vi "Project Target Application.vi"(8 "Error In":errorcluster, 10 "Project Name":string, 11 "App In":refnum<vi>) -> (0 "Error Out":errorcluster, 2 "Project Target App":refnum<vi>, 3 "App Out":refnum<vi>)   [LabVIEW 2017, in "Bookmark Manager.lvlib"]
uses:
  Bookmark Manager.lvlib
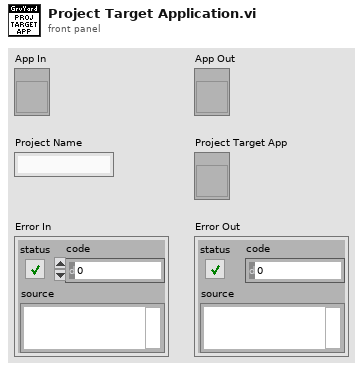
[diagram p1: front panel]
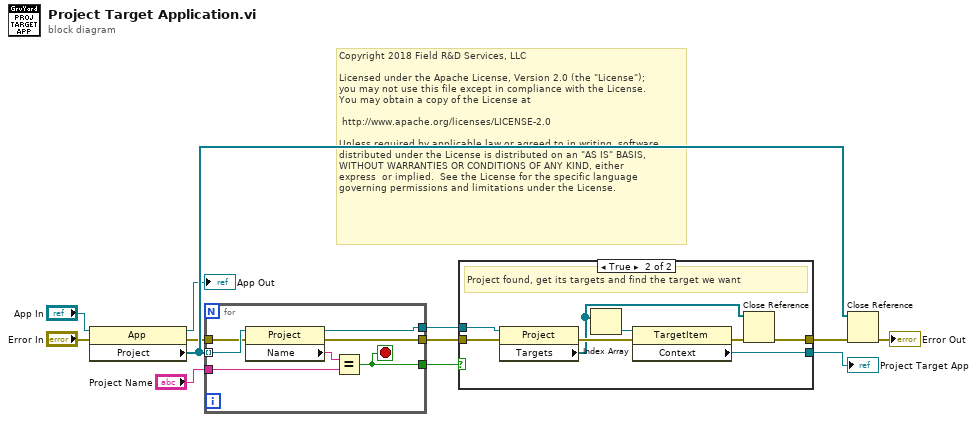
[diagram p0: block diagram]
diagram:
  # "Copyright 2018 Field R&D Services, LLC\n\nLicensed under the Apache License, Version 2.0 (the \"License\");\nyou may not use this file except in compliance with the License.\nYou may obtain a copy of the License at\n\n\thttp://www.apache.org/licenses/LICENSE-2.0\n\nUnless required by applicable law or agreed to in writing, software\ndistributed under the License is distributed on an \"AS IS\" BASIS,\nWITHOUT WARRANTIES OR CONDITIONS OF ANY KIND, either \nexpress  or implied.  See the License for the specific language \ngoverning permissions and limitations under the License."
  n1 = property class="App"(reference="App In", error in="Error In") -> (reference out=→"App Out":refnum<vi>, error out=w5:errorcluster, "Project"=w12:refnum<vi>[])
  n2 = for {
    tunnel: w12 -> [w19] mode=indexing
    tunnel: w5 -> [w18]
    tunnel: "Project Name" -> [w16]
    tunnel: [w15] -> w9
    tunnel: [w14] -> w8
    tunnel: [w13] -> w7
    stop <- w13 stop-if-true
    n3 = property class="Project"(reference=w19, error in=w18) -> (reference out=w15:refnum<vi>, error out=w14:errorcluster, "Name"=w17:string)
    n4 = Equal?(x=w17, y=w16) -> (x = y?=w13:bool)
  }
  n5 = case shown="True" w7 {
    tunnel: w8 -> [w20 w28]
    tunnel: [w20 w22] -> w10
    tunnel: w9 -> [_ w27]
    tunnel: [_ w24] -> w2
    frame False {
      # "Project not found, weird"
    }
    frame True {
      # "Project found, get its targets and find the target we want"
      n6 = property class="Project"(reference=w27, error in=w28) -> (error out=w25:errorcluster, "Targets"=w21:refnum<vi>[])  [unwired: 1 out]
      n7 = Index Array(array=w21) -> (element=w26:refnum<vi>)  [unwired: 1 in]
      n8 = property class="TargetItem"(reference=w26, error in=w25) -> (error out=w23:errorcluster, "Context"=w24:refnum<vi>)  [unwired: 1 out]
      n9 = Close Reference(reference=w21, error in (no error)=w23) -> (error out=w22:errorcluster)
    }
  }
  "Project Target App" <- w2
  n10 = Close Reference(reference=w12, error in (no error)=w10) -> (error out=→"Error Out":errorcluster)
